vi "Delete DVR.vi"(8 "Error In":errorcluster, 11 "DVR Ref Array":T1[](array[typedef])) -> (0 "Error out":errorcluster)   [LabVIEW 2019, in "Arithemetic Operation.lvclass"]
doc: "The VI deletes the data value references of the class data."
uses:
  Arithemetic Operation.lvclass
  Typedef/DVR Ref.ctl
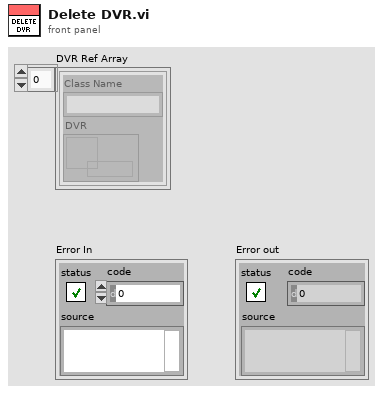
[diagram p1: front panel]
types:
  T1 = typedef "DVR Ref.ctl" = cluster{"Class Name":string, "DVR":refnum<data-value>}
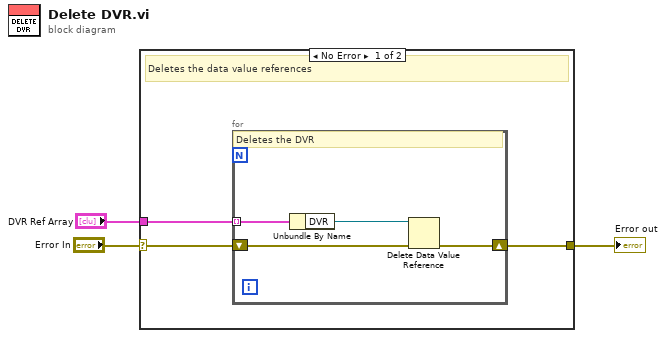
[diagram p0: block diagram]
diagram:
  n1 = case shown="No Error" "Error In" {
    selector: "Error In" -> [w5 w11]
    tunnel: "DVR Ref Array" -> [w6 _]
    tunnel: [w4 w11] -> w1
    frame No Error {
      # "Deletes the data value references"
      n2 = for {
        tunnel: w6 -> [w10] mode=indexing
        shift-right: [w7] -> w4
        shift-left: w5 -> [w8]
        # "Deletes the DVR"
        n3 = Unbundle By Name(w10) -> ("DVR"=w9:refnum<data-value>)
        n4 = Delete Data Value Reference(data value reference=w9, error in=w8) -> (error out=w7:errorcluster)  [unwired: 1 out]
      }
    }
    frame Error {
    }
  }
  "Error out" <- w1
